vi "继保动作转.vi"(1 "动作报告in":bool[](array[boolean])=[FALSE, FALSE, FALSE, FALSE, FALSE, FALSE, FALSE, FALSE, FALSE, FALSE, FALSE, FALSE, FALSE, FALSE, FALSE, FALSE, FALSE, FALSE, FALSE, FALSE, FALSE, FALSE, FALSE, FALSE, FALSE, FALSE]) -> (0 "动作报告out":T1)   [LabVIEW 2015]
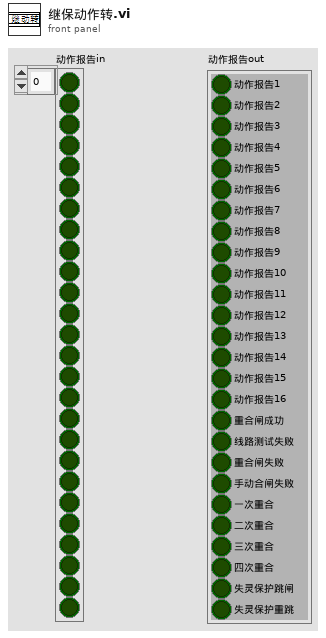
[diagram p1: front panel]
types:
  T1 = cluster{"动作报告1":bool, "动作报告2":bool, "动作报告3":bool, "动作报告4":bool, "动作报告5":bool, "动作报告6":bool, "动作报告7":bool, "动作报告8":bool, "动作报告9":bool, "动作报告10":bool, "动作报告11":bool, "动作报告12":bool, "动作报告13":bool, "动作报告14":bool, "动作报告15":bool, "动作报告16":bool, "重合闸成功":bool, "线路测试失败":bool, "重合闸失败":bool, "手动合闸失败":bool, "一次重合":bool, "二次重合":bool, "三次重合":bool, "四次重合":bool, "失灵保护跳闸":bool, "失灵保护重跳":bool}
  T2 = cluster{"Boolean":bool, "Boolean":bool, "Boolean":bool, "Boolean":bool, "Boolean":bool, "Boolean":bool, "Boolean":bool, "Boolean":bool, "Boolean":bool, "Boolean":bool, "Boolean":bool, "Boolean":bool, "Boolean":bool, "Boolean":bool, "Boolean":bool, "Boolean":bool, "Boolean":bool, "Boolean":bool, "Boolean":bool, "Boolean":bool, "Boolean":bool, "Boolean":bool, "Boolean":bool, "Boolean":bool, "Boolean":bool, "Boolean":bool}
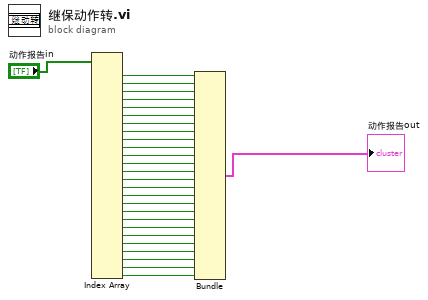
[diagram p0: block diagram]
diagram:
  n1 = Index Array(array="动作报告in") -> (element #1=w27:bool, element #2=w26:bool, element #3=w25:bool, element #4=w24:bool, element #5=w23:bool, element #6=w22:bool, element #7=w21:bool, element #8=w20:bool, element #9=w19:bool, element #10=w18:bool, element #11=w17:bool, element #12=w16:bool, element #13=w15:bool, element #14=w14:bool, element #15=w13:bool, element #16=w12:bool, element #17=w11:bool, element #18=w10:bool, element #19=w9:bool, element #20=w8:bool, element #21=w7:bool, element #22=w6:bool, element #23=w5:bool, element #24=w4:bool, element #25=w3:bool, element #26=w2:bool)  [unwired: 26 in]
  n2 = Bundle("Boolean"=w27, "Boolean"=w26, "Boolean"=w25, "Boolean"=w24, "Boolean"=w23, "Boolean"=w22, "Boolean"=w21, "Boolean"=w20, "Boolean"=w19, "Boolean"=w18, "Boolean"=w17, "Boolean"=w16, "Boolean"=w15, "Boolean"=w14, "Boolean"=w13, "Boolean"=w12, "Boolean"=w11, "Boolean"=w10, "Boolean"=w9, "Boolean"=w8, "Boolean"=w7, "Boolean"=w6, "Boolean"=w5, "Boolean"=w4, "Boolean"=w3, "Boolean"=w2) -> (→"动作报告out":T2)  [unwired: 1 in]
